vi "Write Deadzone.vi"(8 "error in (no error)":errorcluster, 10 "Deadzone":dbl=0.2, 11 "DriverXBoxController in":refnum<class "DriverXBoxController.lvclass">) -> (0 "error out":errorcluster, 3 "DriverXBoxController out":refnum<class "DriverXBoxController.lvclass">)   [LabVIEW 2013, in "DriverXBoxController.lvclass"]
uses:
  DriverXBoxController.lvclass
  DriverXBoxController.lvclass/DriverXBoxController.ctl
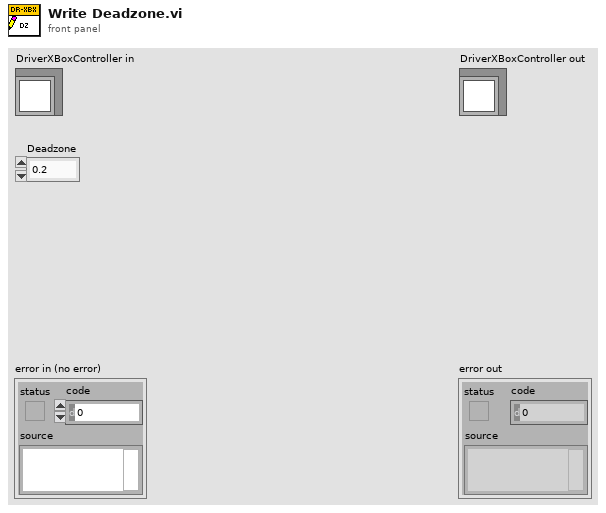
[diagram p1: front panel]
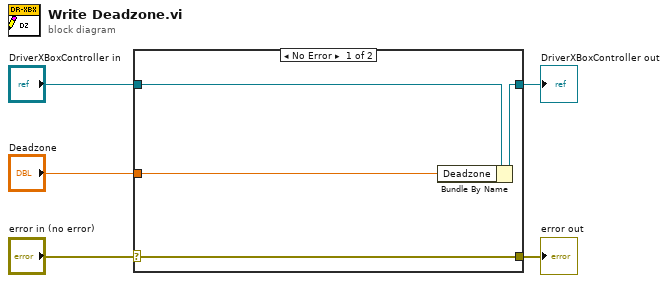
[diagram p0: block diagram]
diagram:
  n1 = case shown="No Error" "error in (no error)" {
    selector: "error in (no error)" -> [w9 w10]
    tunnel: [w9 w10] -> w4
    tunnel: [w7 w11] -> w2
    tunnel: "DriverXBoxController in" -> [w8 w11]
    tunnel: "Deadzone" -> [w6 _]
    frame No Error {
      n2 = Bundle By Name(cluster=w8, "Deadzone"=w6) -> (w7:refnum<class "DriverXBoxController.lvclass">)
    }
    frame Error {
    }
  }
  "error out" <- w4
  "DriverXBoxController out" <- w2
